vi "市电监测变量初始化.vi"(8 "error in (no error)":errorcluster) -> (0 "error out":errorcluster caption="错误输出", 3 "数据":T1)   [LabVIEW 2016, in "环境动力监测库.lvlib" / "自动重合闸库.lvlib"]
uses:
  <vilib>/Utility/config.llb/NI_LVConfig.lvlib
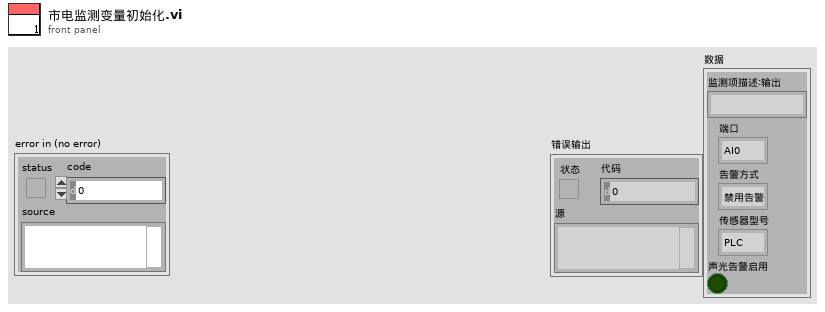
[diagram p1: front panel]
types:
  T1 = cluster{"监测项描述:输出":string, "端口":enum16{"AI0", "AI1", "AI2", "AI3", "AI4", "DI0", "DI1", "DI2", "DI3", "DI4", "DI5", "DI6", "DI7", "DO0", "DO1", "DO2", "DO3", "DO4", "DO5", "DO6", "DO7", "X0", "X1", "X2", "X3", "X4", "X5", "X6", "X7", "X8", "X9", "X10", "X11", "X12", "X13", "X14", "X15", "X16", "X17", "X18", "X19", "X20", "X21", "X22", "X23", "Y0", "Y1", "Y2", "Y3", "Y4", "Y5", "Y6", "Y7", "Y8", "Y9", "Y10", "Y11", "Y12", "Y13", "Y14", "Y15", "Y16", "Y17", "Y18", "Y19", "Y20", "Y21", "Y22", "Y23", "Y24", "Y25", "Y26", "Y27", "Y28", "Y29", "Y30", "Y31", "Y32", "Y33", "Y34", "Y35", "Y36", "Y37", "Y38", "Y39"}, "告警方式":enum32{"禁用告警", "闭合告警", "断开告警"}, "传感器型号":enum16{"PLC", "ZLAN", "ART"}, "声光告警启用":bool}
  T2 = typedef "NI_LVConfig.lvlib/Config Data RefNum.ctl" = refnum<k1>
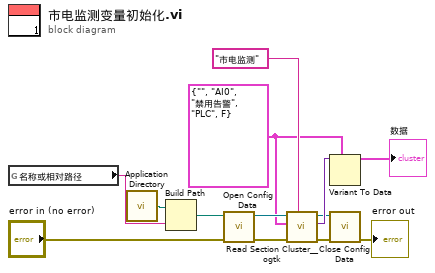
[diagram p0: block diagram]
diagram:
  w2 = T1 {"监测项描述:输出"="", "端口"=enum."AI0", "告警方式"=enum."禁用告警", "传感器型号"=enum."PLC", "声光告警启用"=FALSE} ("簇1输出")
  n1 = global read "内部交互全局变量.vi" "名称或相对路径"() -> (w3:string)
  n2 = call <vilib>:"Application Directory.vi"() -> ("Application Directory"=w9:path)
  n3 = Build Path(base path=w9, name or relative path=w3) -> (appended path=w8:path)
  n4 = call <vilib>:"Open Config Data.vi"("error in (no error)"="error in (no error)", "configuration file path"=w8) -> ("error out"=w7:errorcluster, "refnum"=w6:T2)  [unwired: 7 in, 1 out]
  n5 = call <userlib>:"Read Section Cluster__ogtk.vi"("section (optional)"="市电监测", "error in (no error)"=w7, "Section Formatted Cluster Type"=w2, "refnum"=w6) -> ("error out"=w12:errorcluster, "Section Formatted Cluster"=w13:variant, "dup refnum"=w11:T2)  [unwired: 3 in, 2 out]
  n6 = Variant To Data(type=w2, Variant=w13) -> (data=→"数据":T1)  [unwired: 1 in, 1 out]
  n7 = call <vilib>:"Close Config Data.vi"("error in (no error)"=w12, "refnum"=w11) -> ("error out"=→"error out":errorcluster)  [unwired: 8 in, 1 out]
